vi "ROI_Image_Draw Feret Line.vi"(6 "Pixel Measurements":T4[](array[typedef]) items=["Center of Mass X", "Center of Mass Y", "First Pixel X", "First Pixel Y", "Bounding Rect Left", "Bounding Rect Top", "Bounding Rect Right", "Bounding Rect Bottom", "Max Feret Diameter Start X", "Max Feret Diameter Start Y", "Max Feret Diameter End X", "Max Feret Diameter End Y", "Max Horiz. Segment Length Left", "Max Horiz. Segment Length Right", "Max Horiz. Segment Length Row", "-", "Bounding Rect Width", "Bounding Rect Height", "Bounding Rect Diagonal", "Perimeter", "Convex Hull Perimeter", "Holes' Perimeter", "Max Feret Diameter", "Equivalent Ellipse Major Axis", "Equivalent Ellipse Minor Axis", "Equivalent Ellipse Minor Axis (Feret)", "Equivalent Rect Long Side", "Equivalent Rect Short Side", "Equivalent Rect Diagonal", "Equivalent Rect Short Side (Feret)", "Average Horiz. Segment Length", "Average Vert. Segment Length", "Hydraulic Radius", "Waddel Disk Diameter", "-", "Area", "Holes' Area", "Particle & Holes' Area", "Convex Hull Area", "Image Area", "-", "Number of Holes", "Number of Horiz. Segments", "Number of Vert. Segments", "-", "Orientation", "Max Feret Diameter Orientation", "-", "% Area/Image Area", "% Area/(Particle & Holes' Area)", "Ratio of Equivalent Ellipse Axes", "Ratio of Equivalent Rect Sides", "-", "Elongation Factor", "Compactness Factor", "Heywood Circularity Factor", "Type Factor", "-", "Sum X", "Sum Y", "Sum XX", "Sum XY", "Sum YY", "Sum XXX", "Sum XXY", "Sum XYY", "Sum YYY", "-", "Moment of Inertia XX", "Moment of Inertia XY", "Moment of Inertia YY", "Moment of Inertia XXX", "Moment of Inertia XXY", "Moment of Inertia XYY", "Moment of Inertia YYY", "Norm. Moment of Inertia XX", "Norm. Moment of Inertia XY", "Norm. Moment of Inertia YY", "Norm. Moment of Inertia XXX", "Norm. Moment of Inertia XXY", "Norm. Moment of Inertia XYY", "Norm. Moment of Inertia YYY", "Hu Moment 1", "Hu Moment 2", "Hu Moment 3", "Hu Moment 4", "Hu Moment 5", "Hu Moment 6", "Hu Moment 7"], 8 "error in (no error)":errorcluster, 9 "Particle Measurements (Pixels)":dbl[](array[numeric]), 10 "Circle Data":T3, 11 "Image in":T1) -> (0 "error out":errorcluster, 2 "ROI":T2 {"Contours"."Type" items=["No Selection", "Point", "Line", "Rectangle", "Oval", "Polygon", "Freehand Region", "Annulus", "Unused2", "Unused3", "Broken Line", "Freehand Line", "Rotated Rectangle"]}, 3 "Image out":T1)   [LabVIEW 2014]
uses:
  <vilib>/vision/Image Controls.llb/IMAQ Image.ctl
  <vilib>/vision/NI_Vision_Development_Module.lvlib
panel:
  out "Image for display":T1(plugin-control)
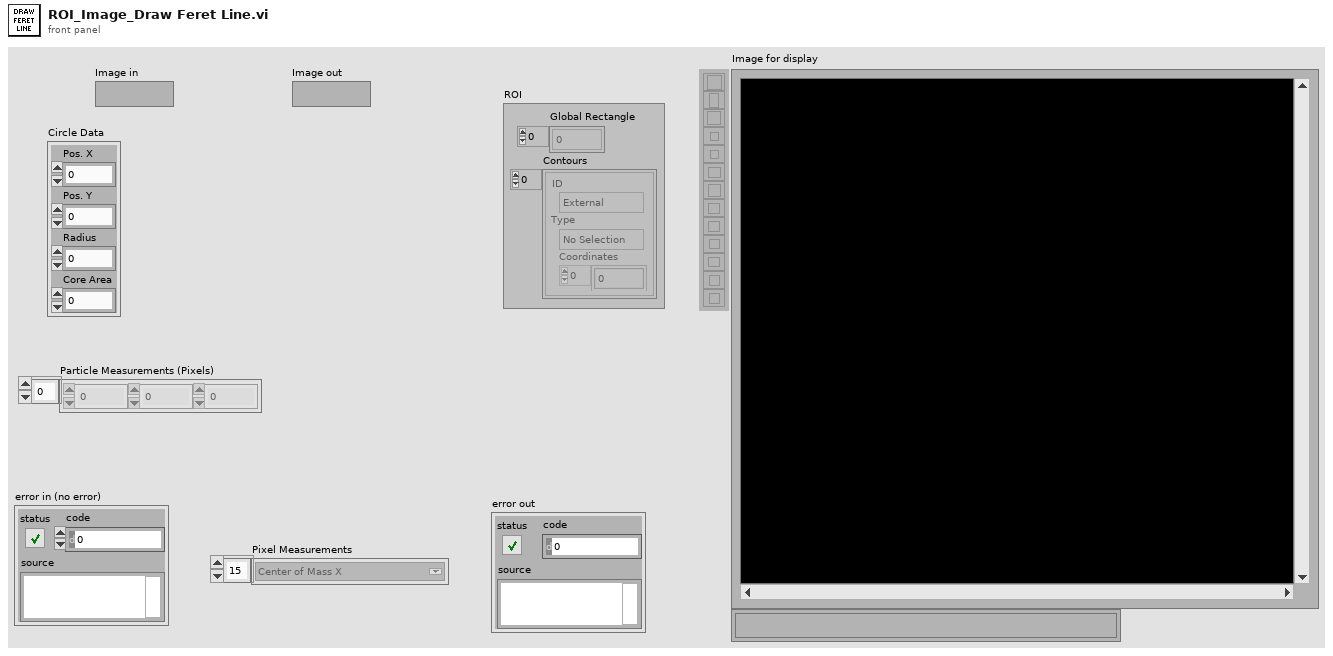
[diagram p1: front panel]
types:
  T1 = typedef "IMAQ Image.ctl" = refnum<image>
  T2 = typedef "ROI Descriptor" = cluster{"Global Rectangle":i32[], "Contours":cluster{"ID":enum32{"External", "Internal"}, "Type":u32, "Coordinates":i32[]}[]}
  T3 = cluster{"Pos. X":i32, "Pos. Y":i32, "Radius":i32, "Core Area":i32}
  T4 = typedef "Particle Parameters" = i32
  T5 = cluster{"Left":i32, "Top":i32, "Right":i32, "Bottom":i32}
  T6 = typedef "enum - StartPt Relative to Circle Center.ctl" = enum16{"X to the Right; Y Below", "X to the Right; Y Above", "X to the Left; Y Below", "X to the Left: Y Above"}
  T7 = cluster{"Point 1":cluster{"X":sgl, "Y":sgl}, "Point 2":cluster{"X":sgl, "Y":sgl}}
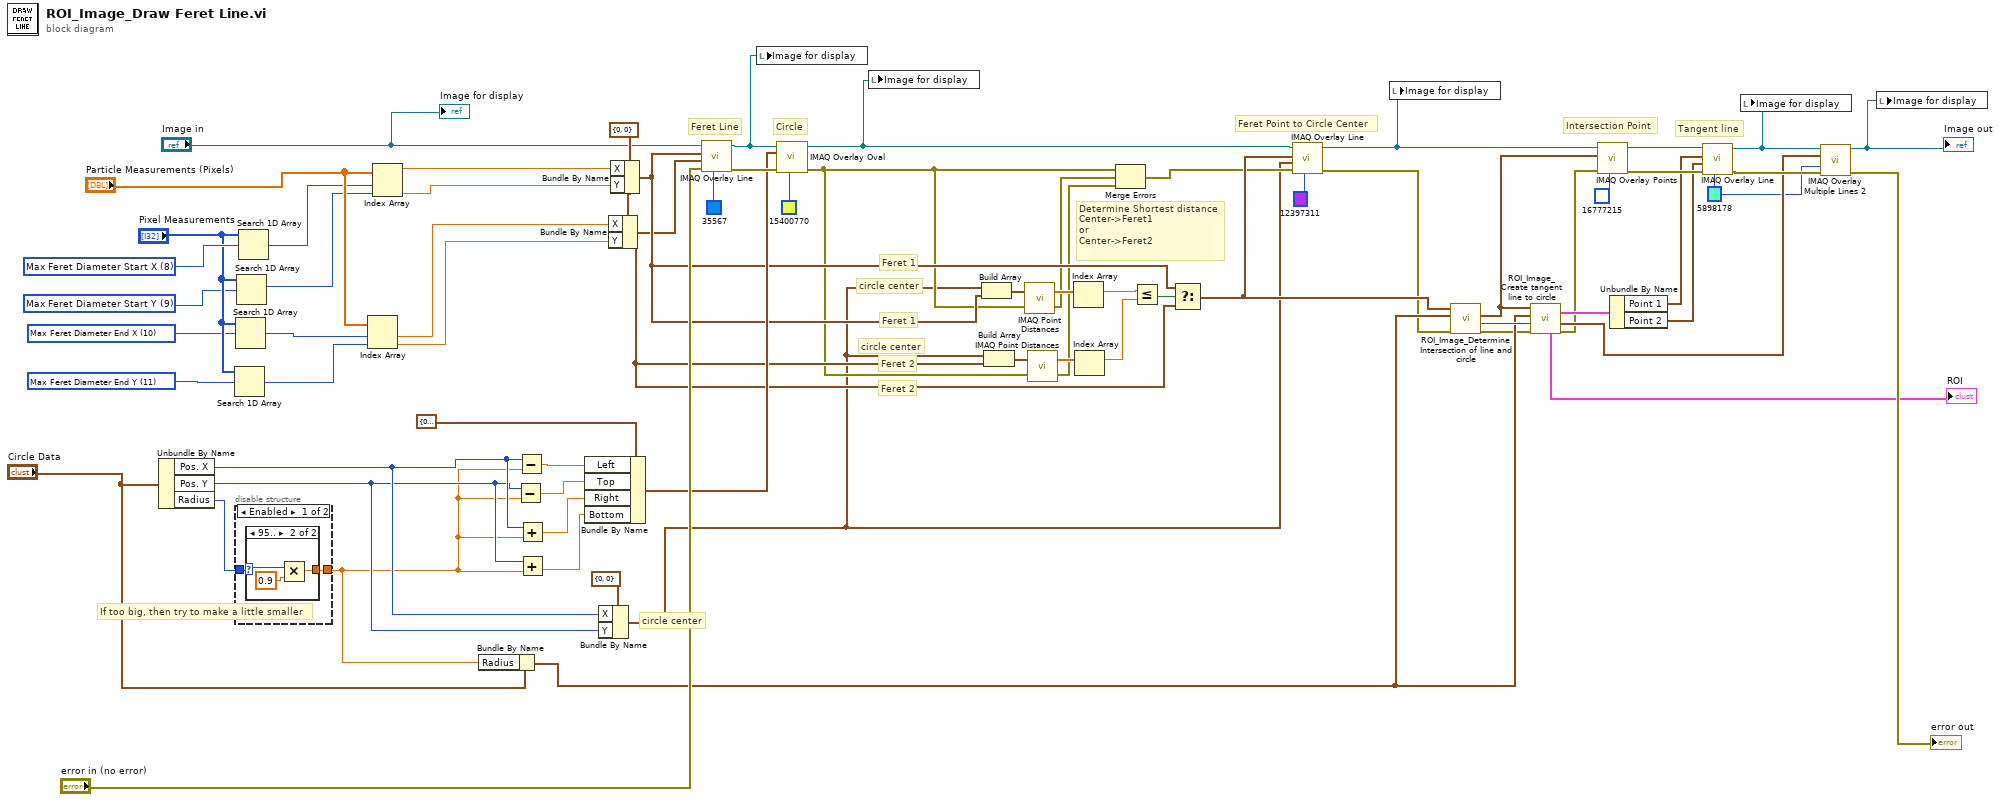
[diagram p0: block diagram]
diagram:
  w25 = u32 5898178 ("Color")
  w70 = cluster{"X":i32, "Y":i32} {"X"=0, "Y"=0} ("Start Point")
  w65 = T4 11 items=["Center of Mass X", "Center of Mass Y", "First Pixel X", "First Pixel Y", "Bounding Rect Left", "Bounding Rect Top", "Bounding Rect Right", "Bounding Rect Bottom", "Max Feret Diameter Start X", "Max Feret Diameter Start Y", "Max Feret Diameter End X", "Max Feret Diameter End Y", "Max Horiz. Segment Length Left", "Max Horiz. Segment Length Right", "Max Horiz. Segment Length Row", "-", "Bounding Rect Width", "Bounding Rect Height", "Bounding Rect Diagonal", "Perimeter", "Convex Hull Perimeter", "Holes' Perimeter", "Max Feret Diameter", "Equivalent Ellipse Major Axis", "Equivalent Ellipse Minor Axis", "Equivalent Ellipse Minor Axis (Feret)", "Equivalent Rect Long Side", "Equivalent Rect Short Side", "Equivalent Rect Diagonal", "Equivalent Rect Short Side (Feret)", "Average Horiz. Segment Length", "Average Vert. Segment Length", "Hydraulic Radius", "Waddel Disk Diameter", "-", "Area", "Holes' Area", "Particle & Holes' Area", "Convex Hull Area", "Image Area", "-", "Number of Holes", "Number of Horiz. Segments", "Number of Vert. Segments", "-", "Orientation", "Max Feret Diameter Orientation", "-", "% Area/Image Area", "% Area/(Particle & Holes' Area)", "Ratio of Equivalent Ellipse Axes", "Ratio of Equivalent Rect Sides", "-", "Elongation Factor", "Compactness Factor", "Heywood Circularity Factor", "Type Factor", "-", "Sum X", "Sum Y", "Sum XX", "Sum XY", "Sum YY", "Sum XXX", "Sum XXY", "Sum XYY", "Sum YYY", "-", "Moment of Inertia XX", "Moment of Inertia XY", "Moment of Inertia YY", "Moment of Inertia XXX", "Moment of Inertia XXY", "Moment of Inertia XYY", "Moment of Inertia YYY", "Norm. Moment of Inertia XX", "Norm. Moment of Inertia XY", "Norm. Moment of Inertia YY", "Norm. Moment of Inertia XXX", "Norm. Moment of Inertia XXY", "Norm. Moment of Inertia XYY", "Norm. Moment of Inertia YYY", "Hu Moment 1", "Hu Moment 2", "Hu Moment 3", "Hu Moment 4", "Hu Moment 5", "Hu Moment 6", "Hu Moment 7"] ("Measurement Parameter")
  w66 = T4 10 items=["Center of Mass X", "Center of Mass Y", "First Pixel X", "First Pixel Y", "Bounding Rect Left", "Bounding Rect Top", "Bounding Rect Right", "Bounding Rect Bottom", "Max Feret Diameter Start X", "Max Feret Diameter Start Y", "Max Feret Diameter End X", "Max Feret Diameter End Y", "Max Horiz. Segment Length Left", "Max Horiz. Segment Length Right", "Max Horiz. Segment Length Row", "-", "Bounding Rect Width", "Bounding Rect Height", "Bounding Rect Diagonal", "Perimeter", "Convex Hull Perimeter", "Holes' Perimeter", "Max Feret Diameter", "Equivalent Ellipse Major Axis", "Equivalent Ellipse Minor Axis", "Equivalent Ellipse Minor Axis (Feret)", "Equivalent Rect Long Side", "Equivalent Rect Short Side", "Equivalent Rect Diagonal", "Equivalent Rect Short Side (Feret)", "Average Horiz. Segment Length", "Average Vert. Segment Length", "Hydraulic Radius", "Waddel Disk Diameter", "-", "Area", "Holes' Area", "Particle & Holes' Area", "Convex Hull Area", "Image Area", "-", "Number of Holes", "Number of Horiz. Segments", "Number of Vert. Segments", "-", "Orientation", "Max Feret Diameter Orientation", "-", "% Area/Image Area", "% Area/(Particle & Holes' Area)", "Ratio of Equivalent Ellipse Axes", "Ratio of Equivalent Rect Sides", "-", "Elongation Factor", "Compactness Factor", "Heywood Circularity Factor", "Type Factor", "-", "Sum X", "Sum Y", "Sum XX", "Sum XY", "Sum YY", "Sum XXX", "Sum XXY", "Sum XYY", "Sum YYY", "-", "Moment of Inertia XX", "Moment of Inertia XY", "Moment of Inertia YY", "Moment of Inertia XXX", "Moment of Inertia XXY", "Moment of Inertia XYY", "Moment of Inertia YYY", "Norm. Moment of Inertia XX", "Norm. Moment of Inertia XY", "Norm. Moment of Inertia YY", "Norm. Moment of Inertia XXX", "Norm. Moment of Inertia XXY", "Norm. Moment of Inertia XYY", "Norm. Moment of Inertia YYY", "Hu Moment 1", "Hu Moment 2", "Hu Moment 3", "Hu Moment 4", "Hu Moment 5", "Hu Moment 6", "Hu Moment 7"] ("Measurement Parameter")
  w67 = T4 9 items=["Center of Mass X", "Center of Mass Y", "First Pixel X", "First Pixel Y", "Bounding Rect Left", "Bounding Rect Top", "Bounding Rect Right", "Bounding Rect Bottom", "Max Feret Diameter Start X", "Max Feret Diameter Start Y", "Max Feret Diameter End X", "Max Feret Diameter End Y", "Max Horiz. Segment Length Left", "Max Horiz. Segment Length Right", "Max Horiz. Segment Length Row", "-", "Bounding Rect Width", "Bounding Rect Height", "Bounding Rect Diagonal", "Perimeter", "Convex Hull Perimeter", "Holes' Perimeter", "Max Feret Diameter", "Equivalent Ellipse Major Axis", "Equivalent Ellipse Minor Axis", "Equivalent Ellipse Minor Axis (Feret)", "Equivalent Rect Long Side", "Equivalent Rect Short Side", "Equivalent Rect Diagonal", "Equivalent Rect Short Side (Feret)", "Average Horiz. Segment Length", "Average Vert. Segment Length", "Hydraulic Radius", "Waddel Disk Diameter", "-", "Area", "Holes' Area", "Particle & Holes' Area", "Convex Hull Area", "Image Area", "-", "Number of Holes", "Number of Horiz. Segments", "Number of Vert. Segments", "-", "Orientation", "Max Feret Diameter Orientation", "-", "% Area/Image Area", "% Area/(Particle & Holes' Area)", "Ratio of Equivalent Ellipse Axes", "Ratio of Equivalent Rect Sides", "-", "Elongation Factor", "Compactness Factor", "Heywood Circularity Factor", "Type Factor", "-", "Sum X", "Sum Y", "Sum XX", "Sum XY", "Sum YY", "Sum XXX", "Sum XXY", "Sum XYY", "Sum YYY", "-", "Moment of Inertia XX", "Moment of Inertia XY", "Moment of Inertia YY", "Moment of Inertia XXX", "Moment of Inertia XXY", "Moment of Inertia XYY", "Moment of Inertia YYY", "Norm. Moment of Inertia XX", "Norm. Moment of Inertia XY", "Norm. Moment of Inertia YY", "Norm. Moment of Inertia XXX", "Norm. Moment of Inertia XXY", "Norm. Moment of Inertia XYY", "Norm. Moment of Inertia YYY", "Hu Moment 1", "Hu Moment 2", "Hu Moment 3", "Hu Moment 4", "Hu Moment 5", "Hu Moment 6", "Hu Moment 7"] ("Measurement Parameter")
  w69 = T4 8 items=["Center of Mass X", "Center of Mass Y", "First Pixel X", "First Pixel Y", "Bounding Rect Left", "Bounding Rect Top", "Bounding Rect Right", "Bounding Rect Bottom", "Max Feret Diameter Start X", "Max Feret Diameter Start Y", "Max Feret Diameter End X", "Max Feret Diameter End Y", "Max Horiz. Segment Length Left", "Max Horiz. Segment Length Right", "Max Horiz. Segment Length Row", "-", "Bounding Rect Width", "Bounding Rect Height", "Bounding Rect Diagonal", "Perimeter", "Convex Hull Perimeter", "Holes' Perimeter", "Max Feret Diameter", "Equivalent Ellipse Major Axis", "Equivalent Ellipse Minor Axis", "Equivalent Ellipse Minor Axis (Feret)", "Equivalent Rect Long Side", "Equivalent Rect Short Side", "Equivalent Rect Diagonal", "Equivalent Rect Short Side (Feret)", "Average Horiz. Segment Length", "Average Vert. Segment Length", "Hydraulic Radius", "Waddel Disk Diameter", "-", "Area", "Holes' Area", "Particle & Holes' Area", "Convex Hull Area", "Image Area", "-", "Number of Holes", "Number of Horiz. Segments", "Number of Vert. Segments", "-", "Orientation", "Max Feret Diameter Orientation", "-", "% Area/Image Area", "% Area/(Particle & Holes' Area)", "Ratio of Equivalent Ellipse Axes", "Ratio of Equivalent Rect Sides", "-", "Elongation Factor", "Compactness Factor", "Heywood Circularity Factor", "Type Factor", "-", "Sum X", "Sum Y", "Sum XX", "Sum XY", "Sum YY", "Sum XXX", "Sum XXY", "Sum XYY", "Sum YYY", "-", "Moment of Inertia XX", "Moment of Inertia XY", "Moment of Inertia YY", "Moment of Inertia XXX", "Moment of Inertia XXY", "Moment of Inertia XYY", "Moment of Inertia YYY", "Norm. Moment of Inertia XX", "Norm. Moment of Inertia XY", "Norm. Moment of Inertia YY", "Norm. Moment of Inertia XXX", "Norm. Moment of Inertia XXY", "Norm. Moment of Inertia XYY", "Norm. Moment of Inertia YYY", "Hu Moment 1", "Hu Moment 2", "Hu Moment 3", "Hu Moment 4", "Hu Moment 5", "Hu Moment 6", "Hu Moment 7"] ("Measurement Parameter")
  # "Feret 1"
  # "Feret 2"
  # "circle center"
  # "Feret 2"
  # "Feret 1"
  # "circle center"
  # "circle center"
  # "Tangent line"
  # "Feret Point to Circle Center"
  # "Determine Shortest distance\nCenter->Feret1\nor \nCenter->Feret2"
  # "Intersection Point"
  # "Circle"
  # "Feret Line"
  n1 = Unbundle By Name("Circle Data") -> ("Pos. X"=w47:i32, "Pos. Y"=w46:i32, "Radius"=w21:i32)
  n2 = Search 1D Array(1D array="Pixel Measurements", element=w65) -> (index of element=w5:i32)  [unwired: 1 in]
  n3 = Search 1D Array(1D array="Pixel Measurements", element=w66) -> (index of element=w6:i32)  [unwired: 1 in]
  n4 = disable-structure shown="Enabled" {
    disable-tunnel: w21 -> [w72 w77]
    disable-tunnel: [w71 w77] -> w20
    frame Enabled {
      # "If too big, then try to make a little smaller"
      n5 = case shown="95.." w72 {
        selector: w72 -> [w73 w75]
        tunnel: [w73 w76] -> w71
        frame 0, Default {
        }
        frame 95.. {
          n6 = Multiply(x=w75, y=0.9) -> (x*y=w76:dbl)
        }
      }
    }
    frame Disabled {
    }
  }
  n7 = Search 1D Array(1D array="Pixel Measurements", element=w67) -> (index of element=w3:i32)  [unwired: 1 in]
  n8 = Search 1D Array(1D array="Pixel Measurements", element=w69) -> (index of element=w4:i32)  [unwired: 1 in]
  n9 = Index Array(array="Particle Measurements (Pixels)", index #1=w6, index #2=w5) -> (element #1=w61:dbl, element #2=w60:dbl)
  n10 = Index Array(array="Particle Measurements (Pixels)", index #1=w4, index #2=w3) -> (element #1=w64:dbl, element #2=w63:dbl)
  n11 = Bundle By Name(cluster="Circle Data", "Radius"=w20) -> (w22:T3)
  n12 = Subtract(x=w46, y=w20) -> (x-y=w53:dbl)
  n13 = Subtract(x=w47, y=w20) -> (x-y=w54:dbl)
  n14 = Add(x=w47, y=w20) -> (x+y=w52:dbl)
  n15 = Add(x=w46, y=w20) -> (x+y=w51:dbl)
  n16 = Bundle By Name(cluster=T5 {"Left"=0, "Top"=0, "Right"=0, "Bottom"=0} ("Bounding Rectangle"), "Left"=w54, "Top"=w53, "Right"=w52, "Bottom"=w51) -> (w50:T5)
  n17 = Bundle By Name(cluster=cluster{"X":i32, "Y":i32} {"X"=0, "Y"=0} ("Point"), "X"=w47, "Y"=w46) -> (w7:cluster{"X":i32, "Y":i32})
  n18 = Bundle By Name(cluster=w70, "X"=w61, "Y"=w60) -> (w37:cluster{"X":i32, "Y":i32})
  n19 = Bundle By Name(cluster=w70, "X"=w64, "Y"=w63) -> (w38:cluster{"X":i32, "Y":i32})
  n20 = call "IMAQ Overlay Line"("Color"=u32 35567, "error in (no error)"="error in (no error)", "End Point"=w37, "Start Point"=w38, "Image"="Image in") -> ("error out"=w57:errorcluster, "Image Out"=w11:T1)  [unwired: 5 in]
  n21 = local write "Image for display"(w11) -> ()
  n22 = call "IMAQ Overlay Oval"("Color"=u32 15400770, "error in (no error)"=w57, "Bounding Rectangle"=w50, "Image"=w11) -> ("error out"=w19:errorcluster, "Image Out"=w10:T1)  [unwired: 6 in]
  n23 = local write "Image for display"(w10) -> ()
  n24 = Build Array(w7, w38) -> (w45:cluster{"X":i32, "Y":i32}[])
  n25 = Build Array(w7, w37) -> (w44:cluster{"X":i32, "Y":i32}[])
  n26 = call "IMAQ Point Distances"("Points"=w45, "error in (no error)"=w19) -> ("Distances"=w43:sgl[], "error out"=w15:errorcluster)  [unwired: 3 in]
  n27 = call "IMAQ Point Distances"("Points"=w44, "error in (no error)"=w19) -> ("Distances"=w42:sgl[], "error out"=w14:errorcluster)  [unwired: 3 in]
  n28 = Index Array(array=w43) -> (element=w41:sgl)  [unwired: 1 in]
  n29 = Index Array(array=w42) -> (element=w40:sgl)  [unwired: 1 in]
  n30 = Merge Errors(w19, w15, w14) -> (w16:errorcluster)
  n31 = Less Or Equal?(x=w41, y=w40) -> (x <= y?=w39:bool)
  n32 = Select(t=w38, s=w39, f=w37) -> (s? t:f=w35:cluster{"X":i32, "Y":i32})
  n33 = call "IMAQ Overlay Line"("Color"=u32 12397311, "error in (no error)"=w16, "End Point"=w7, "Start Point"=w35, "Image"=w10) -> ("error out"=w1:errorcluster, "Image Out"=w2:T1)  [unwired: 5 in]
  n34 = local write "Image for display"(w2) -> ()
  n35 = call "ROI_Image_Determine Intersection of line and circle.vi"("error in (no error)"=w1, "Circles Data"=w22, "Start Point"=w35) -> ("error out"=w18:errorcluster, "Orient rel to center"=w24:T6, "Intersection point"=w13:cluster{"X":i32, "Y":i32})  [unwired: 6 in]
  n36 = call "ROI_Image_Create tangent line to circle.vi"("error in (no error)"=w18, "Orient rel to center"=w24, "Circles Data"=w22, "Intersection Point"=w13) -> ("error out"=w17:errorcluster, "Line End Points"=w26:cluster{"X":dbl, "Y":dbl}[], "Tangent Line"=w31:T7, "ROI"=→"ROI":T2)  [unwired: 4 in]
  n37 = call "IMAQ Overlay Points"("Color"=u32 16777215, "error in (no error)"=w17, "Point"=w13, "Image"=w2) -> ("error out"=w33:errorcluster, "Image Out"=w32:T1)  [unwired: 6 in]
  n38 = Unbundle By Name(w31) -> ("Point 1"=w30:cluster{"X":sgl, "Y":sgl}, "Point 2"=w29:cluster{"X":sgl, "Y":sgl})
  n39 = call "IMAQ Overlay Line"("Color"=w25, "error in (no error)"=w33, "End Point"=w29, "Start Point"=w30, "Image"=w32) -> ("error out"=w28:errorcluster, "Image Out"=w9:T1)  [unwired: 5 in]
  n40 = local write "Image for display"(w9) -> ()
  n41 = call "IMAQ Overlay Multiple Lines 2"("Image"=w9, "Line End Points"=w26, "Color"=w25, "error in (no error)"=w28) -> ("Image Out"=w8:T1, "error out"=→"error out":errorcluster)  [unwired: 10 in]
  "Image out" <- w8
  n42 = local write "Image for display"(w8) -> ()
  "Image for display" <- "Image in"
